vi "Secure Server Example.vi"() -> ()   [LabVIEW 2020]
doc: "A simple Secure WebSockets Server demo."
uses:
  <vilib>/MediaMongrels Ltd/WebSockets/Sockets/VISA TCP Socket/VISA TCP.lvclass
  C:/Program Files (x86)/National Instruments/LabVIEW 2020/vi.lib/MediaMongrels Ltd/WebSockets/Sockets/Socket/Socket.lvclass
  <vilib>/MediaMongrels Ltd/WebSockets/Sockets/VISA TCP Listener/VISA TCP Listener.lvclass
  <vilib>/MediaMongrels Ltd/WebSockets/WebSockets/WebSocket Server/WebSocket Server.lvclass
  Secure Sockets Addon/Secure Sockets Addon.lvlib
panel:
  in  "stop":bool
  out "Read Data":string
  in  "Cert Chain":path
  in  "PK Password":string
  in  "PK Certificate":path
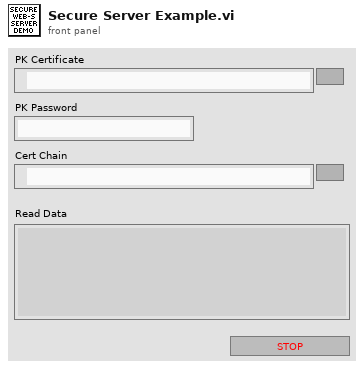
[diagram p1: front panel]
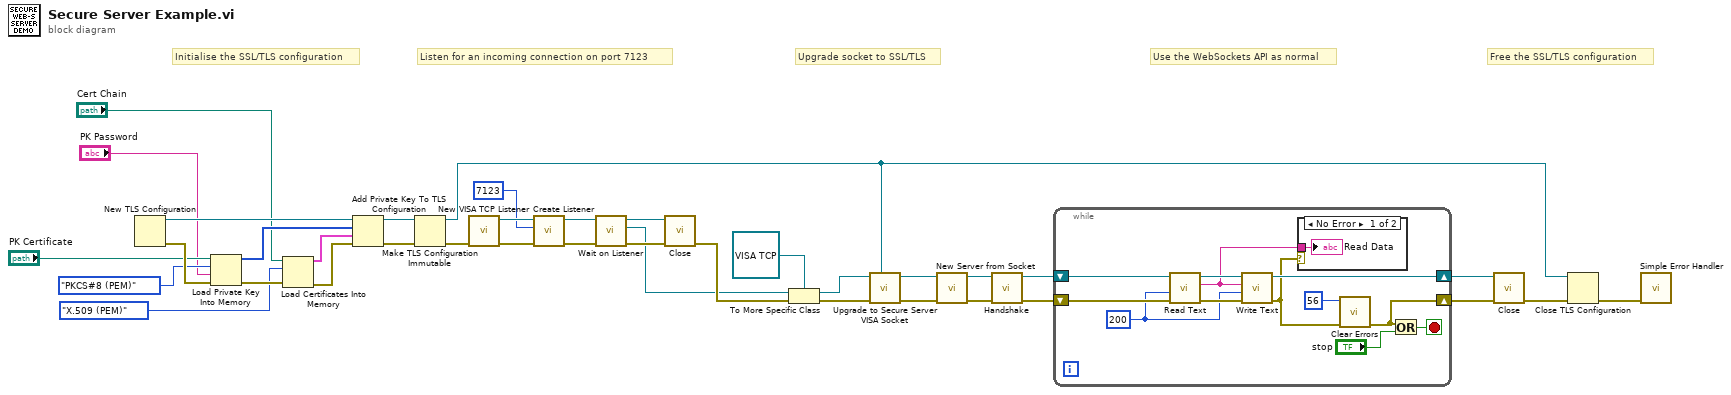
[diagram p0: block diagram]
diagram:
  # "Free the SSL/TLS configuration"
  # "Use the WebSockets API as normal"
  # "Upgrade socket to SSL/TLS"
  # "Listen for an incoming connection on port 7123"
  # "Initialise the SSL/TLS configuration"
  n1 = New TLS Configuration() -> (0:w24:errorcluster, 3:w25:refnum<k36>)  [unwired: 2 in]
  n2 = Load Private Key Into Memory(8:w24, 9:"PK Password", 10:enum32{"PKCS#8 (PEM)", "PKCS#8 (DER)"}."PKCS#8 (PEM)" ("format"), 11:"PK Certificate") -> (0:w23:errorcluster, 3:w28:u8[])
  n3 = Load Certificates Into Memory(8:w23, 10:enum32{"X.509 (PEM)"}."X.509 (PEM)" ("format"), 11:"Cert Chain") -> (0:w26:errorcluster, 3:w27:cluster{"certificate":u8[]}[])
  n4 = Add Private Key To TLS Configuration(8:w26, 9:w27, 10:w28, 11:w25) -> (0:w15:errorcluster, 3:w2:refnum<k36>)
  n5 = Make TLS Configuration Immutable(8:w15, 11:w2) -> (0:w3:errorcluster, 3:w1:refnum<k36>)
  n6 = call <vilib>:"New VISA TCP Listener.vi"("error in (no error)"=w3) -> ("error out"=w36:errorcluster, "VISA TCP Listener out"=w37:refnum<class "VISA TCP Listener.lvclass">)  [unwired: 9 in]
  n7 = call-dynamic "Create Listener.vi"("error in (no error)"=w36, "Port"=u16 7123, "VISA TCP Listener in"=w37) -> ("error out"=w34:errorcluster, "VISA TCP Listener out"=w35:refnum<class "VISA TCP Listener.lvclass">)  [unwired: 7 in]
  n8 = call-dynamic "Wait on Listener.vi"("error in (no error)"=w34, "VISA TCP Listener in"=w35) -> ("error out"=w32:errorcluster, "Socket out"=w6:refnum<class "Socket.lvclass">, "VISA TCP Listener out"=w31:refnum<class "VISA TCP Listener.lvclass">)  [unwired: 7 in]
  n9 = call-dynamic "Close.vi"("error in (no error)"=w32, "VISA TCP Listener in"=w31) -> ("error out"=w8:errorcluster)  [unwired: 9 in]
  n10 = To More Specific Class(target class=refnum<class "VISA TCP.lvclass"> refnum ("VISA TCP Socket in"), reference=w6, error in=w8) -> (specific class reference=w4:refnum<class "VISA TCP.lvclass">, error out=w7:errorcluster)
  n11 = call "Upgrade to Secure Server VISA Socket.vi"("immutable TLS Configuration"=w1, "error in (no error)"=w7, "VISA TCP Socket in"=w4) -> ("error out"=w10:errorcluster, "Secure Server VISA Socket out"=w9:refnum<class "VISA TCP.lvclass">)  [unwired: 6 in, 1 out]
  n12 = call <vilib>:"New Server from Socket.vi"("error in (no error)"=w10, "Socket"=w9) -> ("error out"=w29:errorcluster, "WebSocket Server out"=w30:refnum<class "WebSocket Server.lvclass">)  [unwired: 8 in]
  n13 = call-dynamic "Handshake.vi"("error in (no error)"=w29, "WebSocket Connection in"=w30) -> ("error out"=w17:errorcluster, "WebSocket Connection out"=w16:refnum<class "WebSocket Server.lvclass">)  [unwired: 8 in]
  n14 = while {
    shift-right: [w47] -> w12
    shift-left: w16 -> [w49]
    shift-right: [w41] -> w11
    shift-left: w17 -> [w48]
    stop <- w46 stop-if-true
    w42 = 200 ("timeout ms (5000)")
    n15 = call-dynamic "Read Text.vi"("error in (no error)"=w48, "timeout ms (5000)"=w42, "WebSocket in"=w49) -> ("error out"=w45:errorcluster, "Data"=w38:string, "WebSocket out"=w44:refnum<class "WebSocket Server.lvclass">)  [unwired: 6 in]
    n16 = call-dynamic "Write Text.vi"("error in (no error)"=w45, "timeout ms (5000)"=w42, "String Data"=w38, "WebSocket in"=w44) -> ("error out"=w39:errorcluster, "WebSocket out"=w47:refnum<class "WebSocket Server.lvclass">)  [unwired: 6 in]
    n17 = case shown="No Error" w39 {
      tunnel: w38 -> [w50 _]
      frame No Error {
        "Read Data" <- w50
      }
      frame Error {
      }
    }
    n18 = call <vilib>:"Clear Errors.vi"("error in (no error)"=w39, "specific error code to clear (0: all)"=56) -> ("error out"=w41:errorcluster)  [unwired: 4 in, 1 out]
    n19 = Or(x=w41, y="stop") -> (x .or. y?=w46:bool)
  }
  n20 = call-dynamic "Close.vi"("error in (no error)"=w11, "WebSocket in"=w12) -> ("error out"=w14:errorcluster)  [unwired: 9 in]
  n21 = Close TLS Configuration(8:w14, 11:w1) -> (0:w13:errorcluster)
  n22 = call <vilib>:"Simple Error Handler.vi"("error in (no error)"=w13) -> ()  [unwired: 4 in, 5 out]
